vi "Bode Plot.vi"() -> ()   [LabVIEW 2018]
panel:
  out "Bode":cluster{dbl[], dbl[]}(graph)
  out "Output Data":dbl[][](array[numeric])
  in  "Input Data":dbl[][](array[numeric])=[[0.0, 2.0, 0.0], [0.5, 2.0, 0.0], [1.0, 2.0, 0.0], [1.5, 2.0, 0.0], [2.0, 2.0, 0.0], [2.5, 2.0, 0.0], [3.0, 2.0, 0.0]]
  # "Controls Board"
  # "Bode Plot"
  # "f (Hz)"
  # "Amp (V)"
  # "Vel (rad/s)"
  # "Gain \n(rad/s/V)"
  # "f (Hz)"
  # "Gain (dB)"
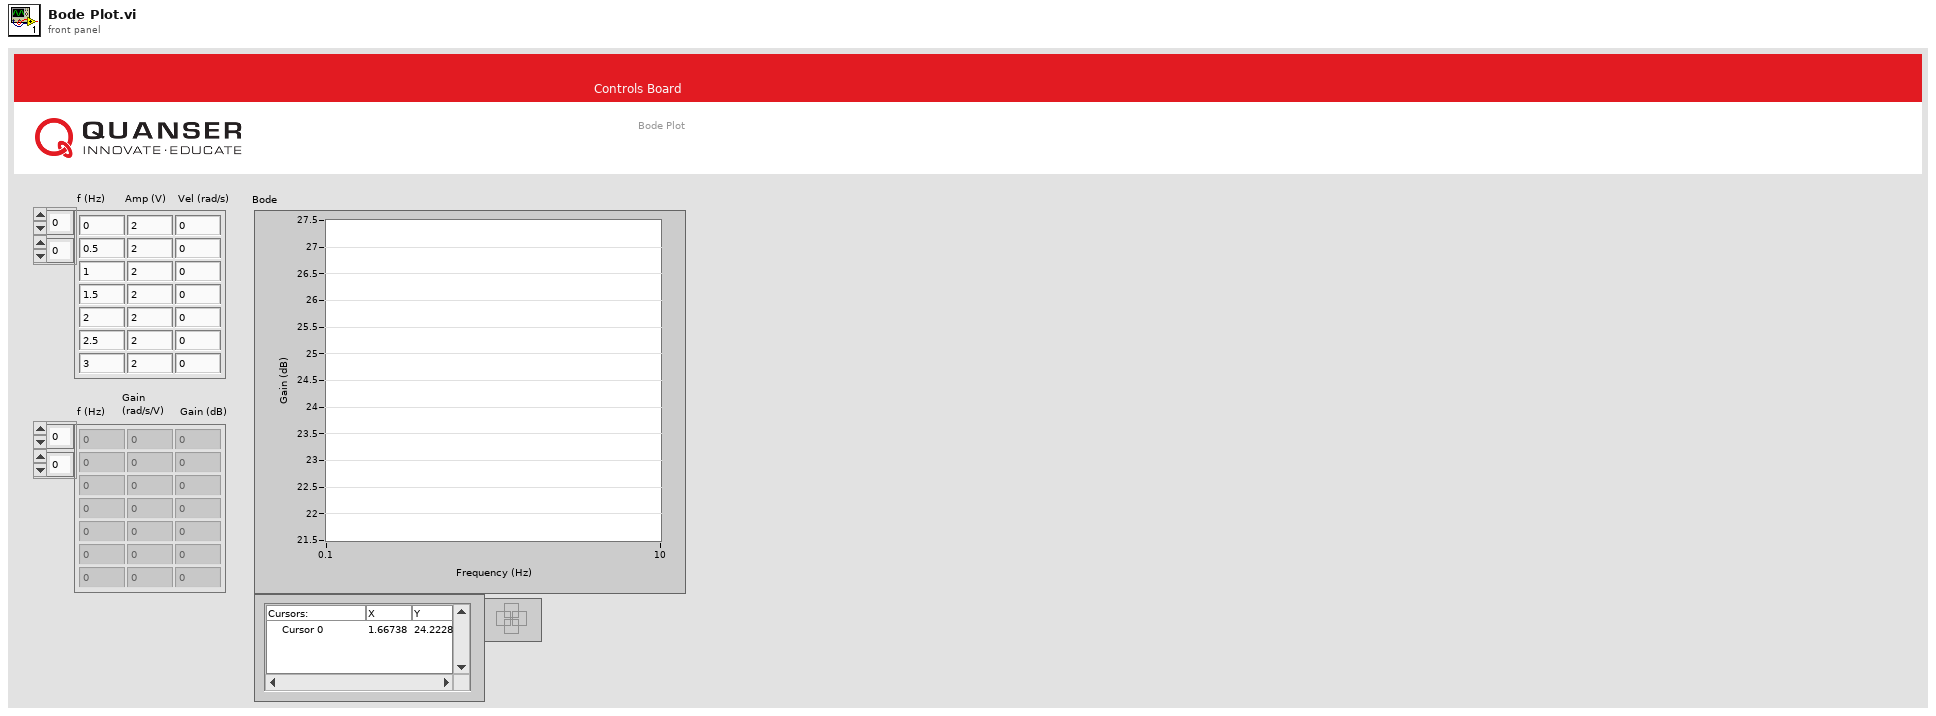
[diagram p1: front panel]
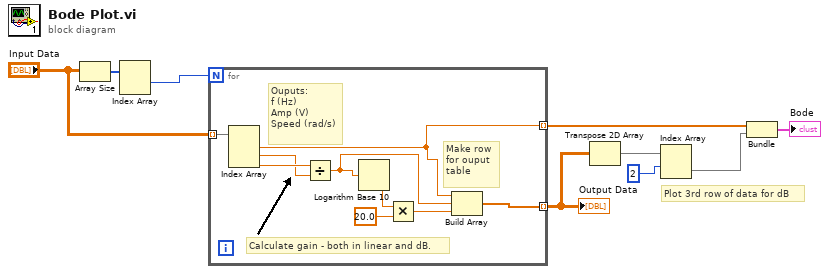
[diagram p0: block diagram]
diagram:
  # "Plot 3rd row of data for dB"
  n1 = Array Size(array="Input Data") -> (size(s)=w9:i32[])
  n2 = Index Array(array=w9) -> (element #1=w8:i32)  [unwired: 2 in, 1 out]
  n3 = for {
    N: w8 -> [_]
    tunnel: "Input Data" -> [w18] mode=indexing
    tunnel: [w17] -> w5 mode=indexing
    tunnel: [w10] -> w3 mode=indexing
    # "Calculate gain - both in linear and dB."
    # "Make row\nfor ouput\ntable"
    # "Ouputs: \nf (Hz)\nAmp (V)\nSpeed (rad/s)"
    n4 = Index Array(array=w18) -> (element #1=w10:dbl, element #2=w15:dbl, element #3=w16:dbl)  [unwired: 3 in]
    n5 = Divide(x=w16, y=w15) -> (x/y=w11:dbl)
    n6 = Logarithm Base 10(1:w11) -> (0:w14:dbl)
    n7 = Multiply(x=w14, y=20.0) -> (x*y=w12:dbl)
    n8 = Build Array(w10, w11, w12) -> (w17:dbl[])
  }
  "Output Data" <- w5
  n9 = Transpose 2D Array(2D array=w5) -> (transposed array=w4:dbl[][])
  n10 = Index Array(array=w4, index (row)=2) -> (element=w2:dbl[])  [unwired: 1 in]
  n11 = Bundle(w3, w2) -> (→"Bode":cluster{dbl[], dbl[]})  [unwired: 1 in]
